vi "Encrypts.vi"(8 "error in (no error)":errorcluster caption="entrée d'erreur (pas d'erreur)", 11 "Cryptographic Hash_SHA256 en entrée":refnum<class "Cryptographic Hash_SHA256_File.lvclass">) -> (0 "error out":errorcluster caption="sortie d'erreur", 3 "Cryptographic Hash_SHA256 en sortie":refnum<class "Cryptographic Hash_SHA256_File.lvclass">)   [LabVIEW 2020, in "Library Cryptographic Hash.lvlib" / "Cryptographic Hash_SHA256_File.lvclass"]
uses:
  Cryptographic Hash_SHA256_File.lvclass
  C:/Users/ngarcin/OneDrive - Altyor/Standard TB/Class/Cryptographic Hash/Cryptographic Hash (Default)/Cryptographic Hash (Default).lvclass
  C:/Users/ngarcin/OneDrive - Altyor/Standard TB/Class/Cryptographic Hash/Cryptographic Hash_SHA256/Cryptographic Hash_SHA256.lvclass
  Cryptographic Hash_SHA256_File.lvclass/Cryptographic Hash_SHA256_File.ctl
  Commun VI/Library Commun.lvlib
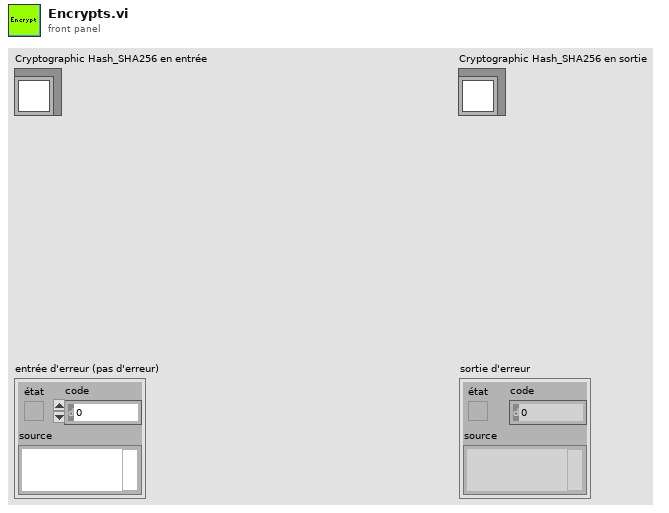
[diagram p1: front panel]
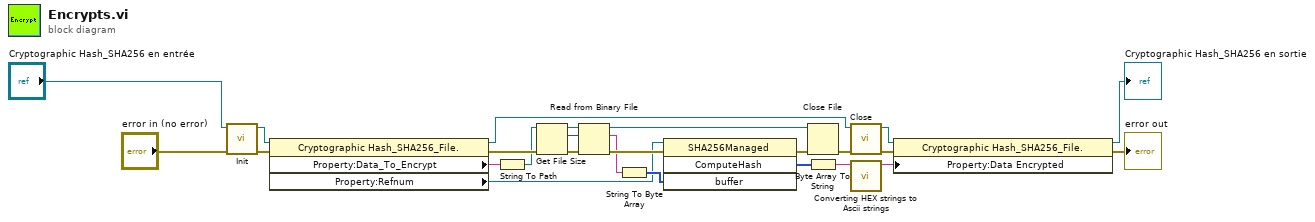
[diagram p0: block diagram]
diagram:
  n1 = call-dynamic "Init.vi"("error in (no error)"="error in (no error)", "Cryptographic Hash_SHA256 en entrée"="Cryptographic Hash_SHA256 en entrée") -> ("error out"=w15:errorcluster, "Cryptographic Hash_SHA256 en sortie"=w16:refnum<class "Cryptographic Hash_SHA256_File.lvclass">)  [unwired: 8 in]
  n2 = property class="Cryptographic Hash_SHA256_File."(reference=w16, error in=w15) -> (reference out=w11:refnum<class "Cryptographic Hash_SHA256_File.lvclass">, error out=w14:errorcluster, "Property:Data_To_Encrypt"=w9:string, "Property:Refnum"=w3:refnum<k24>)
  n3 = String To Path(string=w9) -> (path=w8:path)
  n4 = Get File Size(file=w8, error in=w14) -> (refnum out=w19:refnum<file>, size (in bytes)=w18:i64, 0:w20:errorcluster)
  n5 = Read from Binary File(8:w20, 10:w18, 11:w19) -> (0:w25:errorcluster, 2:w24:string, 3:w21:refnum<file>)  [unwired: 3 in, 1 out]
  n6 = String To Byte Array(string=w24) -> (unsigned byte array=w23:u8[])
  n7 = invoke class="SHA256Managed" method="ComputeHash"(reference=w3, error in=w25, "buffer"=w23) -> (error out=w7:errorcluster, "ComputeHash"=w22:u8[])  [unwired: 1 in, 2 out]
  n8 = Close File(refnum=w21, error in=w7) -> (error out=w12:errorcluster)  [unwired: 1 out]
  n9 = Byte Array To String(unsigned byte array=w22) -> (string=w2:string)
  n10 = call-dynamic "Close.vi"("error in (no error)"=w12, "Cryptographic Hash_SHA256 en entrée"=w11) -> ("error out"=w5:errorcluster, "Cryptographic Hash_SHA256 en sortie"=w10:refnum<class "Cryptographic Hash_SHA256_File.lvclass">)  [unwired: 8 in]
  n11 = call "Converting HEX strings to Ascii strings.vi"("chaîne IN"=w2) -> ("Chaîne OUT"=w1:string)  [unwired: 9 in, 1 out]
  n12 = property class="Cryptographic Hash_SHA256_File."(reference=w10, error in=w5, "Property:Data Encrypted"=w1) -> (reference out=→"Cryptographic Hash_SHA256 en sortie":refnum<class "Cryptographic Hash_SHA256_File.lvclass">, error out=→"error out":errorcluster)
